vi "U3 Stream AIN with Timers & Counters.vi"() -> ()   [LabVIEW 2021]
panel:
  out "UD Backlog [%]":dbl format="%.2f"
  out "U3 Backlog [%]":dbl format="%.2f"
  in  "Reset Timer1/Counter0":bool
  out "Combined Counter Data":u32[](array[numeric])
  out "# Scans Read":i32
  out "# of iterations":i32
  out "Data":dbl[][](array[numeric]) format="%.3f"
  in  "Scan Rate (Hz)":dbl=1000.0 format="%.3f"
  in  "FirstFound":bool=TRUE
  in  "stop":bool
  in  "Address":string="1"
  out "Error Message":string
  # "This example streams AIN1, Timer1 (duty cycle input on\nFIO5), Counter1 (FIO6), and the FIO/EIO digital inputs.\n\nTimer0 is configured as 16-bit PWM output (FIO4).  Frequency\nis 40.6 Hz and duty cycle is 25%.\n\nFor testing, short FIO4 to FIO5 and FIO6.\n\nStreams using the SLEEP wait mode.  Streaming\nrequires U3 hardware revision 1.21."
  # "AIN1               TMR1 (LSW)         TMR1 (MSW)    CNT (LSW)        CNT(MSW)        FIO/EIO"
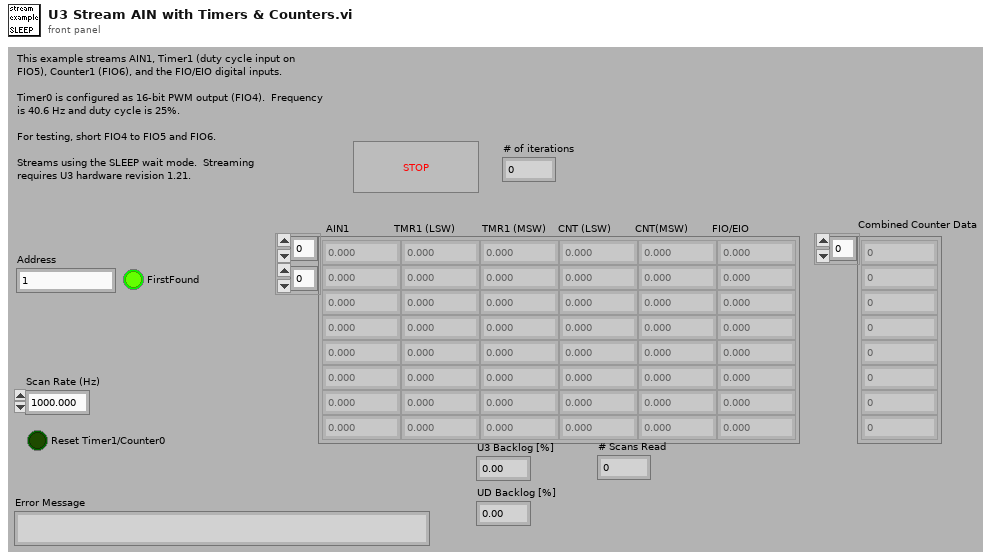
[diagram p1: front panel]
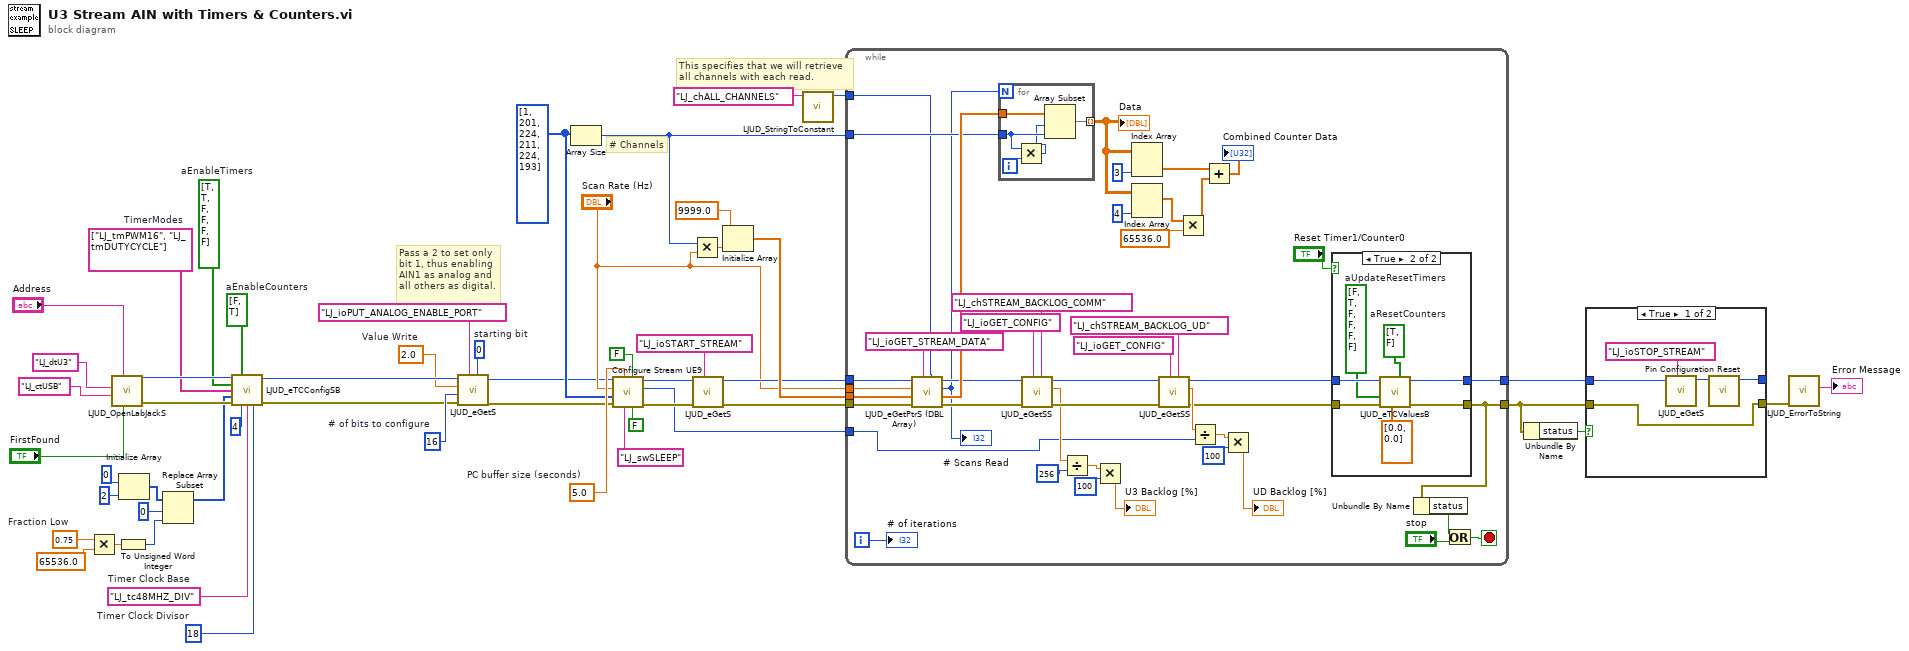
[diagram p0: block diagram]
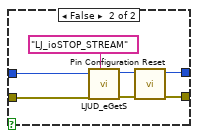
[diagram p3: hidden frame]
diagram:
  w6 = 16  # # of bits to configure
  w8 = 0  # starting bit
  w9 = 2.0  # Value Write
  w14 = 18  # Timer Clock Divisor
  w15 = "LJ_tc48MHZ_DIV"  # Timer Clock Base
  w18 = bool[] [FALSE, TRUE]  # aEnableCounters
  w20 = 0.75  # Fraction Low
  w16 = string[] ["LJ_tmPWM16", "LJ_tmDUTYCYCLE"]  # TimerModes
  w17 = bool[] [TRUE, TRUE, FALSE, FALSE, FALSE, FALSE]  # aEnableTimers
  w30 = i32[] [1, 201, 224, 211, 224, 193] ("Channels")
  w39 = 5.0  # PC buffer size (seconds)
  # "Pass a 2 to set only\nbit 1, thus enabling\nAIN1 as analog and\nall others as digital."
  # "# Channels"
  # "This specifies that we will retrieve\nall channels with each read."
  n1 = Multiply(x=w20, y=65536.0) -> (x*y=w22:dbl)
  n2 = call "LJUD_OpenLabJackS.vi"("FirstFound"="FirstFound", "Address"="Address", "ConnectionType"="LJ_ctUSB", "DeviceType"="LJ_dtU3") -> ("error out"=w28:errorcluster, "Handle"=w29:i32)  [unwired: 5 in, 1 out]
  n3 = To Unsigned Word Integer(number=w22) -> (unsigned 16bit integer=w21:u16)
  n4 = Initialize Array(u16 0 ("PWM Timer Value"), 2 ("Dimension Size")) -> (w24:u16[])
  n5 = Replace Array Subset(array=w24, new element=w21, index=0 ("Index")) -> (w19:u16[])
  n6 = call "LJUD_eTCConfigSB.vi"("Handle In"=w29, "aEnableCounters"=w18, "aEnableTimers"=w17, "aTimerModes"=w16, "aTimerValues"=w19, "error in"=w28, "TCPinOffset"=4, "TimerClockBase"=w15, "TimerClockDivisor"=w14) -> ("Handle Out"=w10:i32, "error out"=w3:errorcluster)  [unwired: 5 in]
  n7 = call "LJUD_eGetS.vi"("Channel"=w8, "IOType"="LJ_ioPUT_ANALOG_ENABLE_PORT", "error in"=w3, "x1"=w6, "Value Write"=w9, "Handle In"=w10) -> ("error out"=w4:errorcluster, "Handle Out"=w5:i32)  [unwired: 3 in, 1 out]
  n8 = Array Size(array=w30) -> (size(s)=w43:i32)
  n9 = call "Configure Stream UE9.vi"("External Scan Trigger"=FALSE, "Scan Clock Output"=FALSE, "Wait Mode"="LJ_swSLEEP" ("Wait Mode (2)"), "PC buffer size (seconds)"=w39, "error in"=w4, "Scan List"=w30, "Scan Rate (Hz)"="Scan Rate (Hz)", "Handle In"=w5) -> ("error out"=w48:errorcluster, "PC buffer size (samples)"=w11:i32, "Handle Out"=w49:i32)  [unwired: 1 in]
  n10 = Multiply(x=w43, y="Scan Rate (Hz)") -> (x*y=w46:dbl)
  n11 = call "LJUD_eGetS.vi"("IOType"="LJ_ioSTART_STREAM", "error in"=w48, "Handle In"=w49) -> ("error out"=w47:errorcluster, "Handle Out"=w36:i32)  [unwired: 6 in, 1 out]
  n12 = Initialize Array(9999.0, w46) -> (w44:dbl[])
  n13 = call "LJUD_StringToConstant.vi"("String"="LJ_chALL_CHANNELS") -> ("Constant Number"=w31:i32)  [unwired: 9 in, 1 out]
  n14 = while {
    tunnel: w11 -> [w55]
    tunnel: w31 -> [w82]
    tunnel: [w71] -> w34
    tunnel: [w70] -> w41
    tunnel: w43 -> [w88]
    tunnel: w44 -> [w91]
    tunnel: "Scan Rate (Hz)" -> [w89]
    tunnel: w47 -> [w93]
    tunnel: w36 -> [w94]
    i -> [w87]
    stop <- w81 stop-if-true
    n15 = call "LJUD_eGetPtrS (DBL Array).vi"("Channel"=w82, "IOType"="LJ_ioGET_STREAM_DATA", "error in"=w93, "DBL Array Write"=w91, "Value"=w89, "Handle In"=w94) -> ("error out"=w85:errorcluster, "DBL Array Read"=w90:dbl[], "Value"=w80:i32, "Handle Out"=w86:i32)  [unwired: 2 in]
    "# Scans Read" <- w80
    n16 = for {
      N: w80 -> [_]
      tunnel: w90 -> [w110]
      tunnel: w88 -> [w109]
      tunnel: [w106] -> w79 mode=indexing
      i -> [w108]
      n17 = Multiply(x=w109, y=w108) -> (x*y=w107:i32)
      n18 = Array Subset(array=w110, index=w107, length=w109) -> (w106:dbl[])
    }
    "Data" <- w79
    n19 = call "LJUD_eGetSS.vi"("Channel"="LJ_chSTREAM_BACKLOG_COMM", "IOType"="LJ_ioGET_CONFIG", "error in"=w85, "Handle In"=w86) -> ("error out"=w62:errorcluster, "Value Read"=w56:dbl, "Handle Out"=w63:i32)  [unwired: 5 in]
    n20 = Divide(x=w56, y=256) -> (x/y=w57:dbl)
    n21 = Multiply(x=w57, y=100) -> (x*y=→"U3 Backlog [%]":dbl)
    n22 = Index Array(array=w79, index (col)=3 ("Disabled Index (col)")) -> (element=w75:dbl[])  [unwired: 1 in]
    n23 = Index Array(array=w79, index (col)=4 ("Disabled Index (col)")) -> (element=w76:dbl[])  [unwired: 1 in]
    n24 = call "LJUD_eGetSS.vi"("Channel"="LJ_chSTREAM_BACKLOG_UD", "IOType"="LJ_ioGET_CONFIG", "error in"=w62, "Handle In"=w63) -> ("error out"=w61:errorcluster, "Value Read"=w64:dbl, "Handle Out"=w60:i32)  [unwired: 5 in]
    n25 = Multiply(x=w76, y=65536.0) -> (x*y=w74:dbl[])
    n26 = Divide(x=w64, y=w55) -> (x/y=w65:dbl)
    n27 = Add(x=w75, y=w74) -> (x+y=→"Combined Counter Data":dbl[])
    n28 = Multiply(x=w65, y=100) -> (x*y=→"UD Backlog [%]":dbl)
    n29 = case shown="True" "Reset Timer1/Counter0" {
      tunnel: w61 -> [w98 w105]
      tunnel: w60 -> [w97 w104]
      tunnel: [w98 w103] -> w71
      tunnel: [w97 w102] -> w70
      frame False {
      }
      frame True {
        w101 = bool[] [TRUE, FALSE]  # aResetCounters
        w100 = bool[] [FALSE, TRUE, FALSE, FALSE, FALSE, FALSE]  # aUpdateResetTimers
        n30 = call "LJUD_eTCValuesB.vi"("aResetCounters"=w101, "aTimerValues Write"=dbl[] [0.0, 0.0], "error in"=w105, "aUpdateResetTimers"=w100, "Handle In"=w104) -> ("error out"=w103:errorcluster, "Handle Out"=w102:i32)  [unwired: 3 in, 2 out]
      }
    }
    n31 = Unbundle By Name(w71) -> ("status"=w95:bool)
    n32 = Or(x=w95, y="stop") -> (x .or. y?=w81:bool)
    "# of iterations" <- w87
  }
  n33 = Unbundle By Name(w34) -> ("status"=w33:bool)
  n34 = case shown="True" w33 {
    tunnel: w41 -> [w114 w121]
    tunnel: [w113 w118] -> w2
    tunnel: w34 -> [w113 w120]
    tunnel: [w111 w116] -> _
    frame True {
      n35 = call "LJUD_eGetS.vi"("IOType"="LJ_ioSTOP_STREAM", "Handle In"=w114) -> ("Handle Out"=w112:i32)  [unwired: 7 in, 2 out]
      n36 = call "Pin Configuration Reset.vi"("Handle In"=w112) -> ("Handle Out"=w111:i32)  [unwired: 9 in, 1 out]
    }
    frame False {
      n37 = call "LJUD_eGetS.vi"("IOType"="LJ_ioSTOP_STREAM", "error in"=w120, "Handle In"=w121) -> ("error out"=w119:errorcluster, "Handle Out"=w117:i32)  [unwired: 6 in, 1 out]
      n38 = call "Pin Configuration Reset.vi"("error in"=w119, "Handle In"=w117) -> ("error out"=w118:errorcluster, "Handle Out"=w116:i32)  [unwired: 8 in]
    }
  }
  n39 = call "LJUD_ErrorToString.vi"("error in"=w2) -> ("String"=→"Error Message":string)  [unwired: 10 in]
